vi "Client 3.vi"() -> ()   [LabVIEW 2019, in "RemoteControl.ZMQ.lvclass"]
uses:
  RemoteControl.ZMQ.lvclass
panel:
  in  "milliseconds to wait":u32
  out "Command Sent":string
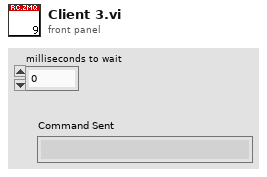
[diagram p1: front panel]
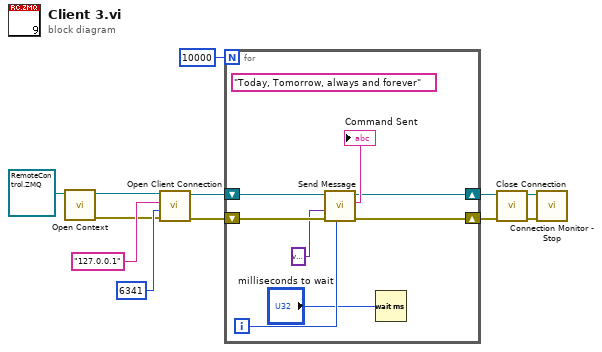
[diagram p0: block diagram]
diagram:
  n1 = call-dynamic "Open Context.vi"("RemoteControl.ZMQ in"=refnum<class "RemoteControl.ZMQ.lvclass"> refnum) -> ("error out"=w1:errorcluster, "RemoteControl.ZMQ out"=w2:refnum<class "RemoteControl.ZMQ.lvclass">)  [unwired: 9 in]
  n2 = call-dynamic "Open Client Connection.vi"("error in (no error)"=w1, "Port"=u16 6341, "address"="127.0.0.1" ("Address"), "RemoteControl.ZMQ in"=w2) -> ("error out"=w10:errorcluster, "RemoteControl.ZMQ out"=w11:refnum<class "RemoteControl.ZMQ.lvclass">)  [unwired: 6 in]
  n3 = for {
    N: 10000 -> [_]
    shift-right: [w16] -> w7
    shift-left: w11 -> [w20]
    shift-right: [w15] -> w6
    shift-left: w10 -> [w19]
    i -> [w14]
    (unwired) "Today, Tomorrow, always and forever" ("Command")
    n4 = call-dynamic "Send Message.vi"("Message ID"=w14, "error in (no error)"=w19, "Data"=variant, "RemoteControl.ZMQ in"=w20) -> ("error out"=w15:errorcluster, "ACK"=→"Command Sent":string, "RemoteControl.ZMQ out"=w16:refnum<class "RemoteControl.ZMQ.lvclass">)  [unwired: 5 in]
    n5 = Wait (ms)(milliseconds to wait="milliseconds to wait") -> ()  [unwired: 1 out]
  }
  n6 = call-dynamic "Close Connection.vi"("error in (no error)"=w6, "RemoteControl.ZMQ in"=w7) -> ("error out"=w8:errorcluster, "RemoteControl.ZMQ out"=w9:refnum<class "RemoteControl.ZMQ.lvclass">)  [unwired: 8 in]
  n7 = call-dynamic "Connection Monitor - Stop.vi"("error in (no error)"=w8, "RemoteControl.ZMQ in"=w9) -> ()  [unwired: 8 in, 2 out]
